vi "XYStage.SetTargetPosition(counts).vi"(8 "error in (no error)":errorcluster, 10 "Target Counts":T2, 11 "XYStage":refnum<class "XYStage.lvclass">) -> (0 "error out":errorcluster, 2 "Real Units Coords":T1, 3 "XYStage out":refnum<class "XYStage.lvclass">)   [LabVIEW 2019, in "XYStage.lvclass"]
doc: "---------------------------------------------------------------\nJKI State Machine Objects™\nhttp://jki.net/state-machine-objects/\nCopyright (C) 2005-2015, JKI <info@jki.net>\nALL RIGHTS RESERVEDJKI State Machine Objects (SMO) 1.0.0.5\nJKI - JKI\nCopyright (c) 2016, JKI"
uses:
  XYStage.lvclass
  Typedefs/(counts)Coords--Cluster.ctl
  Typedefs/(real)Coords--Cluster.ctl
  XYStage.lvclass/XYStage.ctl
panel:
  # "For instructions on how to use the JKI State Machine Objects, examples and video tutorials, visit:\nhttp://jki.net/state-machine-objects/\n\nJKI State Machine Objects™\nhttp://jki.net/state-machine-objects/\nCopyright (C) 2005-2015, JKI <info@jki.net>\nALL RIGHTS RESERVED"
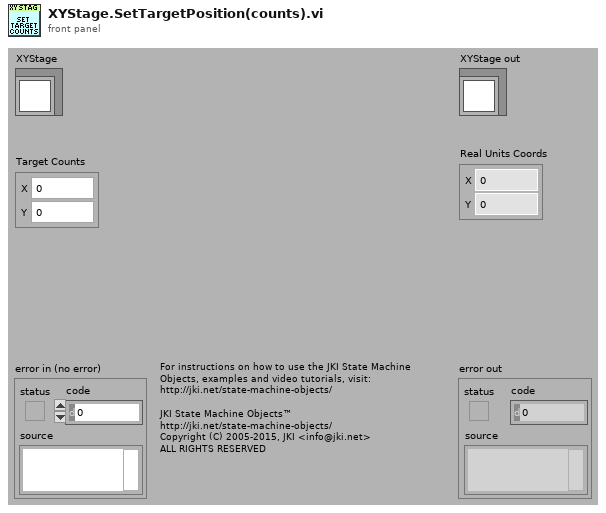
[diagram p1: front panel]
types:
  T1 = typedef "XYStage.lvclass/(real)Coords--Cluster.ctl" = cluster{"X":dbl, "Y":dbl}
  T2 = typedef "XYStage.lvclass/(counts)Coords--Cluster.ctl" = cluster{"X":i32, "Y":i32}
  T3 = typedef "XYStage.lvclass/PrivateData--Ref.ctl" = refnum<data-value>
  T4 = typedef "XYStage.lvclass/PrivateData--Cluster.ctl" = cluster{"Dependencies":T5, "Public Events":T6, "Protected Events":T7, "Private Events":T8, "Configuration":T9, "Target":T10, "Move Parameters":T11}
  T5 = typedef "XYStage.lvclass/Dependencies--Cluster.ctl" = cluster{"Positions":refnum<class "SMO.Dictionary.Variant.lvclass">}
  T6 = typedef "XYStage.lvclass/PublicEvents--Cluster.ctl" = cluster{"MoveComplete":refnum<user-event>, "NewPosition":refnum<user-event>, "UpdatedNamedPosition":refnum<user-event>, "MoveStarted":refnum<user-event>}
  T7 = typedef "XYStage.lvclass/ProtectedEvents--Cluster.ctl" = cluster{"API_Template":refnum<user-event>}
  T8 = typedef "XYStage.lvclass/PrivateEvents--Cluster.ctl" = cluster{"MoveAbsolute":refnum<user-event>, "MoveRelative":refnum<user-event>, "MoveToNamedPosition":refnum<user-event>, "StorePosition":refnum<user-event>, "Home":refnum<user-event>}
  T9 = typedef "XYStage.lvclass/Configuration--Cluster.ctl" = cluster{"Real-World Units":string, "Counts per Unit":dbl}
  T10 = typedef "XYStage.lvclass/TargetPositions--Cluster.ctl" = cluster{"Coords":T1, "Counts":T2}
  T11 = typedef "XYStage.lvclass/MoveParameters--Cluster.ctl" = cluster{"Velocity (units/s)":dbl, "Acceleration (units/s^2)":dbl}
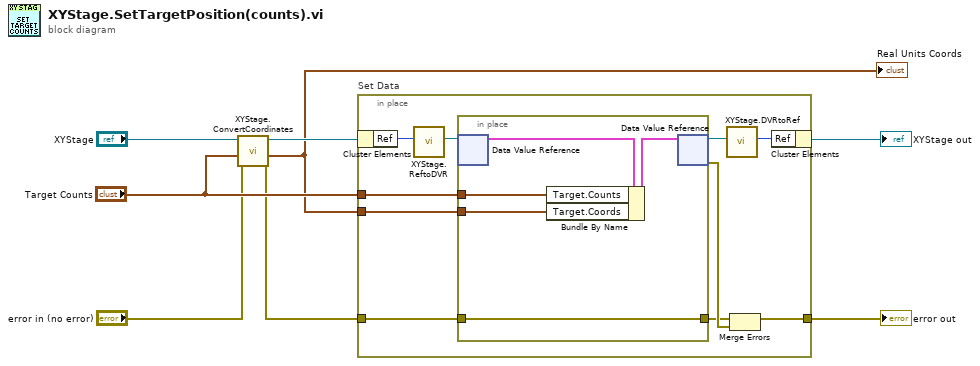
[diagram p0: block diagram]
diagram:
  n1 = call-dynamic "XYStage.ConvertCoordinates.vi"("error in (no error)"="error in (no error)", "Counts"="Target Counts", "XYStage in"="XYStage") -> ("error out"=w2:errorcluster, "Real Units Coords out"=w1:T1, "XYStage out"=w4:refnum<class "XYStage.lvclass">)  [unwired: 5 in, 1 out]
  "Real Units Coords" <- w1
  n2 = in-place "Set Data" {
    in-place-border: w2 -> [w18]
    in-place-border: [w15] -> w8
    in-place-border: "Target Counts" -> [w14]
    in-place-border: w1 -> [w9]
    n3 = in-place-cluster #1(w4) -> ("Ref"=w13:u32)
    n4 = call "XYStage.ReftoDVR.vi"("Ref"=w13) -> ("Ref"=w12:T3)  [unwired: 10 in]
    n5 = in-place {
      in-place-border: w18 -> [w23]
      in-place-border: [w23] -> w16
      in-place-border: w14 -> [w21]
      in-place-border: w9 -> [w20]
      n6 = in-place-dvr #2(w12) -> (w19:T4)  [unwired: 1 out]
      n7 = Bundle By Name(cluster=w19, "Target.Counts"=w21, "Target.Coords"=w20) -> (w22:T4)
      n8 = in-place-dvr #2(w22) -> (w11:T3, w17:errorcluster)
    }
    n9 = call "XYStage.DVRtoRef.vi"("Ref"=w11) -> ("Ref"=w10:u32)  [unwired: 10 in]
    n10 = Merge Errors(w16, w17) -> (w15:errorcluster)
    n11 = in-place-cluster #1("Ref"=w10) -> (→"XYStage out":refnum<class "XYStage.lvclass">)
  }
  "error out" <- w8
